vi "Send Message And Wait For Response.vi"(6 "Name":string, 7 "Priority (normal)":T1, 8 "error in (no error)":errorcluster, 9 "Response Timeout [1000 ms]":i32=1000, 10 "Payload":variant, 11 "Actor API in":refnum<class "Actor API.lvclass">) -> (0 "error out":errorcluster, 3 "Response":variant, 5 "Response Received":bool)   [LabVIEW 2020, in "RTAF.lvlib" / "Actor API.lvclass"]
uses:
  Actor API.lvclass
  <vilib>/event_ctls.llb/usereventprio.ctl
  Actor API.lvclass/Actor API.ctl
  Actor/Message.ctl
  Actor/Actor.lvclass
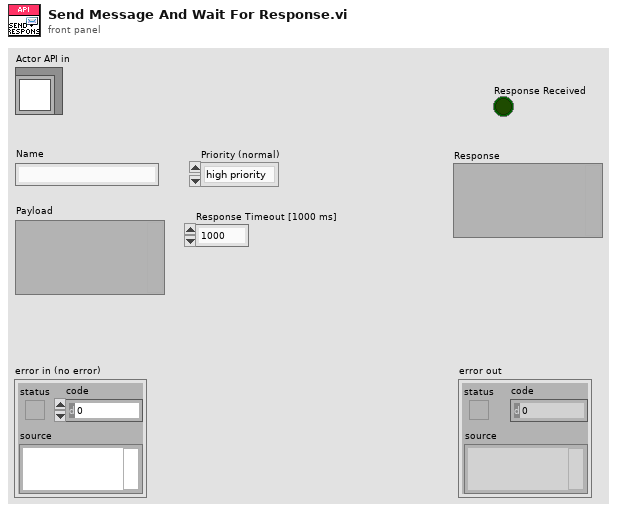
[diagram p1: front panel]
types:
  T1 = typedef "usereventprio.ctl" = enum32{"high priority", "normal priority"}
  T2 = typedef "RTAF.lvlib/Actor.lvclass/Message.ctl" = cluster{"Name":string, "Payload":variant, "Response Channel":refnum<notifier>}
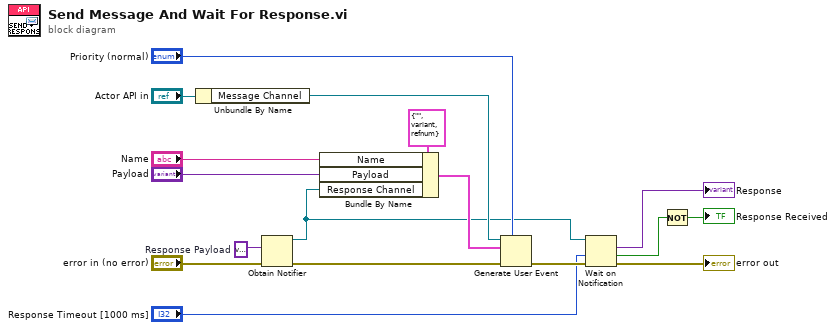
[diagram p0: block diagram]
diagram:
  w7 = variant  # Response Payload
  n1 = Unbundle By Name("Actor API in") -> ("Message Channel"=w15:refnum<user-event>)
  n2 = Obtain Notifier(notification data type=w7, error in (no error)="error in (no error)") -> (notifier out=w6:refnum<notifier>, error out=w2:errorcluster)  [unwired: 2 in, 1 out]
  n3 = Bundle By Name(cluster=T2 {"Name"="", "Payload"=variant, "Response Channel"=refnum} ("Message"), "Name"="Name", "Payload"="Payload", "Response Channel"=w6) -> (w12:T2)
  n4 = Generate User Event(priority (normal)="Priority (normal)", user event=w15, event data cluster=w12, error in=w2) -> (error out=w10:errorcluster)  [unwired: 1 out]
  n5 = Wait on Notification(notifier=w6, timeout in ms (-1)="Response Timeout [1000 ms]", error in (no error)=w10) -> (notification=→"Response":variant, timed out?=w4:bool, error out=→"error out":errorcluster)  [unwired: 1 in, 1 out]
  n6 = Not(x=w4) -> (.not. x?=→"Response Received":bool)
